vi "Queue_Driver.vi"(0 "Name":string, 7 "States_Data[]":T1[](array[typedef]), 11 "Error in":errorcluster, 13 "Operation":T2) -> (8 "State_out":T1, 15 "Error out":errorcluster)   [LabVIEW 2020, in "Automated Teller Machine.lvlib"]
doc: "This Queue Driver holds the State in Sequence which also stores the Value which can pass data from Producer loop to consumer loop"
uses:
  Automated Teller Machine.lvlib
  Type_def/Queue_operations.ctl
  Type_def/Queue_Datatype.ctl
panel:
  # "QUEUE DRIVER"
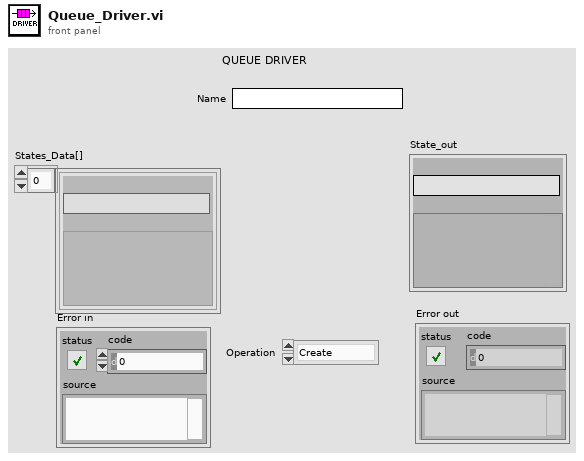
[diagram p1: front panel]
types:
  T1 = typedef "Automated Teller Machine.lvlib/Queue_Datatype.ctl" = cluster{"State":string, "Data":variant}
  T2 = typedef "Automated Teller Machine.lvlib/Queue_operations.ctl" = enum16{"Create", "Enqueue", "Dequeue", "Flush", "Release"}
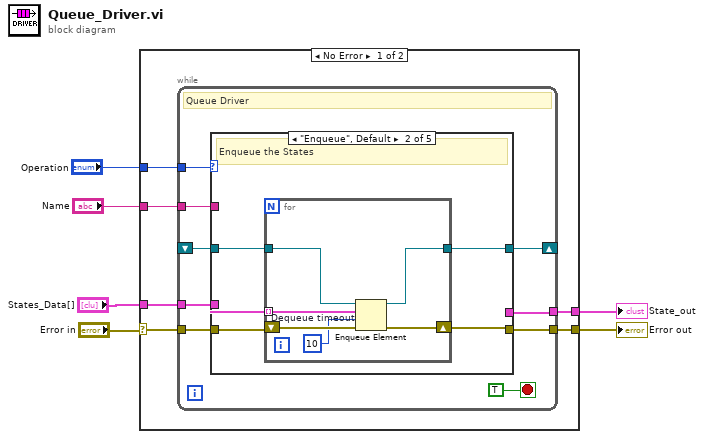
[diagram p0: block diagram]
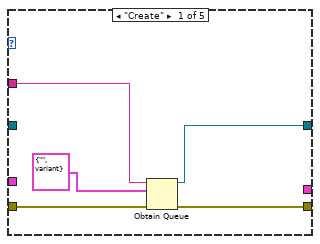
[diagram p2: hidden frame]
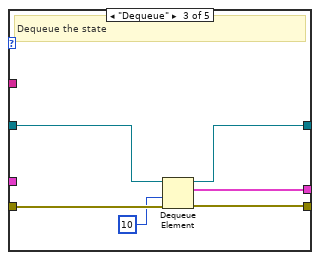
[diagram p3: hidden frame]
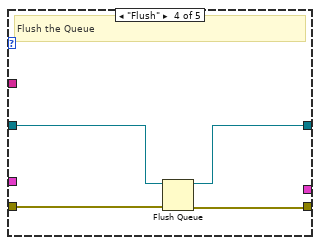
[diagram p4: hidden frame]
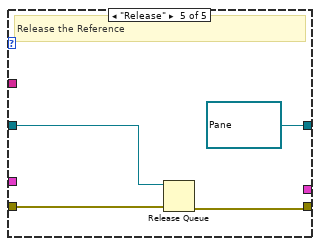
[diagram p5: hidden frame]
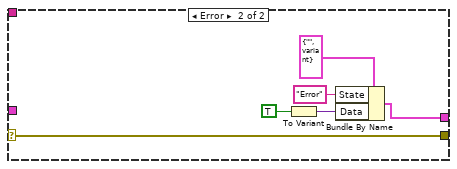
[diagram p6: hidden frame]
diagram:
  n1 = case shown="No Error" "Error in" {
    selector: "Error in" -> [w12 w57]
    tunnel: "Operation" -> [w11 _]
    tunnel: [w10 w57] -> w4
    tunnel: "Name" -> [w9 _]
    tunnel: "States_Data[]" -> [w8 _]
    tunnel: [w7 w55] -> w1
    frame No Error {
      n2 = while {
        tunnel: w12 -> [w20]
        tunnel: w11 -> [w19]
        tunnel: [w18] -> w10
        tunnel: w9 -> [w17]
        shift-right: [w16] -> _
        shift-left: _ -> [w15]
        tunnel: w8 -> [w14]
        tunnel: [w13] -> w7
        stop <- TRUE stop-if-true
        # "Queue Driver"
        n3 = case shown="\"Enqueue\", Default" w19 {
          tunnel: w20 -> [w26 w31 w43 w47 w51]
          tunnel: [w25 w30 w42 w46 w50] -> w18
          tunnel: w17 -> [w24 _ _ _ _]
          tunnel: [w22 w27 w39 w44 refnum<queue> refnum ("queue out")] -> w16
          tunnel: w15 -> [_ w28 w40 w45 w49]
          tunnel: w14 -> [_ w29 _ _ _]
          tunnel: [_ _ w38 _ _] -> w13
          frame "Create" {
            n4 = Obtain Queue(name (unnamed)=w24, element data type=T1 {"State"="", "Data"=variant}, error in (no error)=w26) -> (queue out=w22:refnum<queue>, error out=w25:errorcluster)  [unwired: 2 in, 1 out]
          }
          frame "Enqueue", Default {
            # "Enqueue the States"
            n5 = for {
              shift-right: [w36] -> w30
              shift-left: w31 -> [w37]
              tunnel: w29 -> [w32] mode=indexing
              tunnel: w28 -> [w34]
              tunnel: [w33] -> w27
              w35 = 10  # Dequeue timeout
              n6 = Enqueue Element(queue=w34, element=w32, timeout in ms (-1)=w35, error in (no error)=w37) -> (queue out=w33:refnum<queue>, error out=w36:errorcluster)  [unwired: 1 out]
            }
          }
          frame "Dequeue" {
            # "Dequeue the state"
            n7 = Dequeue Element(queue=w40, timeout in ms (-1)=10, error in (no error)=w43) -> (queue out=w39:refnum<queue>, element=w38:T1, error out=w42:errorcluster)  [unwired: 1 out]
          }
          frame "Flush" {
            # "Flush the Queue"
            n8 = Flush Queue(queue=w45, error in (no error)=w47) -> (queue out=w44:refnum<queue>, error out=w46:errorcluster)  [unwired: 1 out]
          }
          frame "Release" {
            # "Release the Reference"
            n9 = Release Queue(queue=w49, error in (no error)=w51) -> (error out=w50:errorcluster)  [unwired: 1 in, 2 out]
          }
        }
      }
    }
    frame Error {
      n10 = To Variant(anything=TRUE) -> (Variant=w53:variant)
      n11 = Bundle By Name(cluster=T1 {"State"="", "Data"=variant} ("Cluster"), "State"="Error", "Data"=w53) -> (w55:T1)
    }
  }
  "Error out" <- w4
  "State_out" <- w1
